vi "test Compile RaF Data.vi"(8 "error in (no error)":errorcluster, 11 "TestCase in":refnum<class "Routing and Faulting Unit Tests.lvclass">) -> (0 "error out":errorcluster, 3 "TestCase out":refnum<class "Routing and Faulting Unit Tests.lvclass">)   [LabVIEW 2017, in "Routing and Faulting Unit Tests.lvclass"]
uses:
  Routing and Faulting Unit Tests.lvclass
  Shared/Communication Configuration.ctl
  Shared/Routing and Faulting Configuration.ctl
  Shared/Routing Channel Configuration.ctl
  Shared/Value-Connections Map.ctl
  Shared/Connection.ctl
  Shared/Alias Mapping.ctl
  Shared/FIFO Indices.ctl
  Shared/Channel States.ctl
  Shared/Routing State.ctl
  Shared/Compiled.Settings.ctl
  Routing and Faulting Unit Tests.lvclass/Routing and Faulting Unit Tests.ctl
  System Explorer/Get Channel Data in By Channel ID (offline).vi
  Scripting/Switch Scripting.lvlib
  Shared/Routing and Faulting Shared.lvlib
  System Explorer/Routing and Faulting System Explorer.lvlib
panel:
  out "Compiled.Settings":T8
  in  "Save?":bool
  out "Output Filename":string
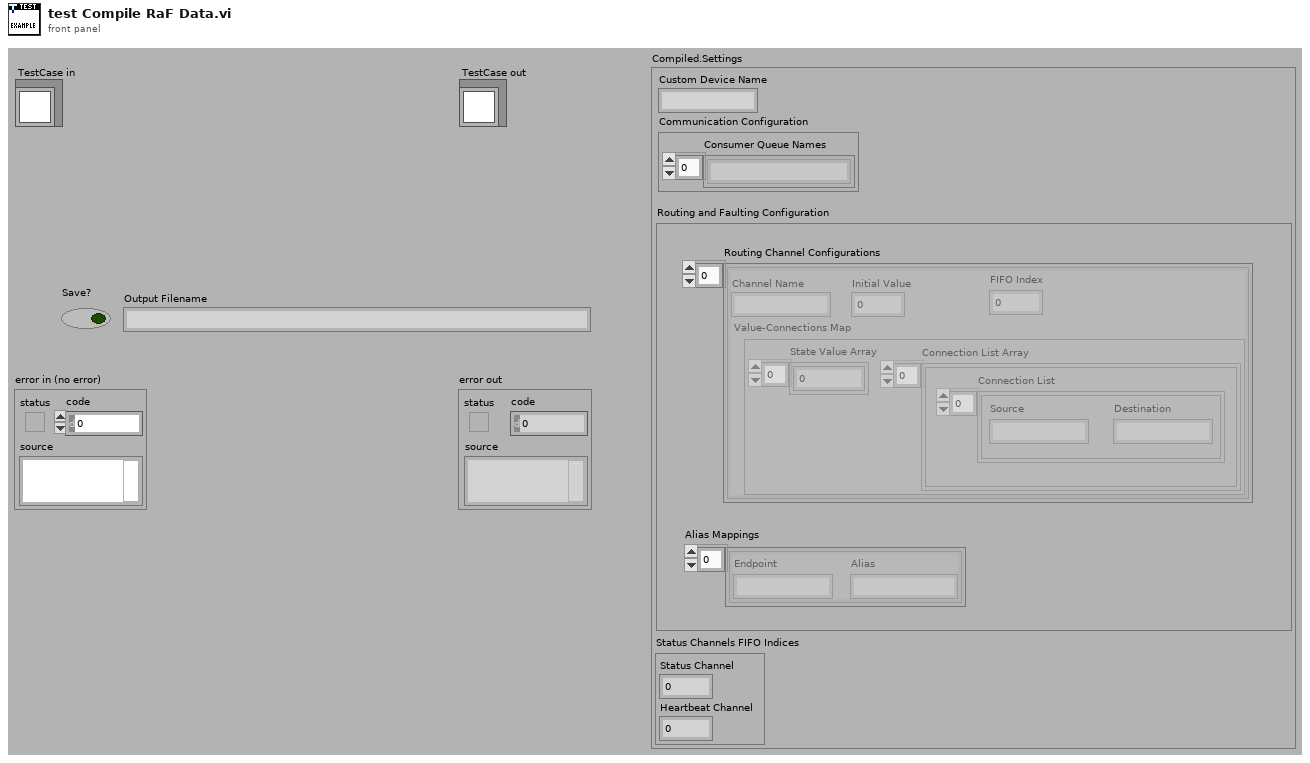
[diagram p1: front panel]
types:
  T1 = typedef "Routing and Faulting Shared.lvlib/Communication Configuration.ctl" = cluster{"Consumer Queue Names":string[]}
  T2 = typedef "Routing and Faulting Shared.lvlib/Routing and Faulting Configuration.ctl" = cluster{"Routing Channel Configurations":T3[], "Alias Mappings":T6[]}
  T3 = typedef "Routing and Faulting Shared.lvlib/Routing Channel Configuration.ctl" = cluster{"Channel Name":string, "Initial Value":dbl, "FIFO Index":i32, "Value-Connections Map":T4}
  T4 = typedef "Routing and Faulting Shared.lvlib/Value-Connections Map.ctl" = cluster{"State Value Array":i32[], "Connection List Array":cluster{"Connection List":T5[]}[]}
  T5 = typedef "Routing and Faulting Shared.lvlib/Connection.ctl" = cluster{"Source":string, "Destination":string}
  T6 = typedef "Routing and Faulting Shared.lvlib/Alias Mapping.ctl" = cluster{"Endpoint":string, "Alias":string}
  T7 = typedef "Routing and Faulting Shared.lvlib/FIFO Indices.ctl" = cluster{"Status Channel":i32, "Heartbeat Channel":i32}
  T8 = cluster{"Custom Device Name":string, "Communication Configuration":T1, "Routing and Faulting Configuration":T2, "Status Channels FIFO Indices":T7}
  T9 = typedef "Routing and Faulting Shared.lvlib/Compiled.Settings.ctl" = cluster{"Custom Device Name":string, "Communication Configuration":T1, "Routing and Faulting Configuration":T2, "Status Channels FIFO Indices":T7}
  T10 = typedef "Routing and Faulting Shared.lvlib/Channel States.ctl" = T11[]
  T11 = typedef "Routing and Faulting Shared.lvlib/Routing State.ctl" = cluster{"Name":string, "Description":string, "Value":i32, "Connection List":T5[]}
  T12 = typedef "Custom Device API.lvlib/Custom Device Item Ref.ctl" = u64
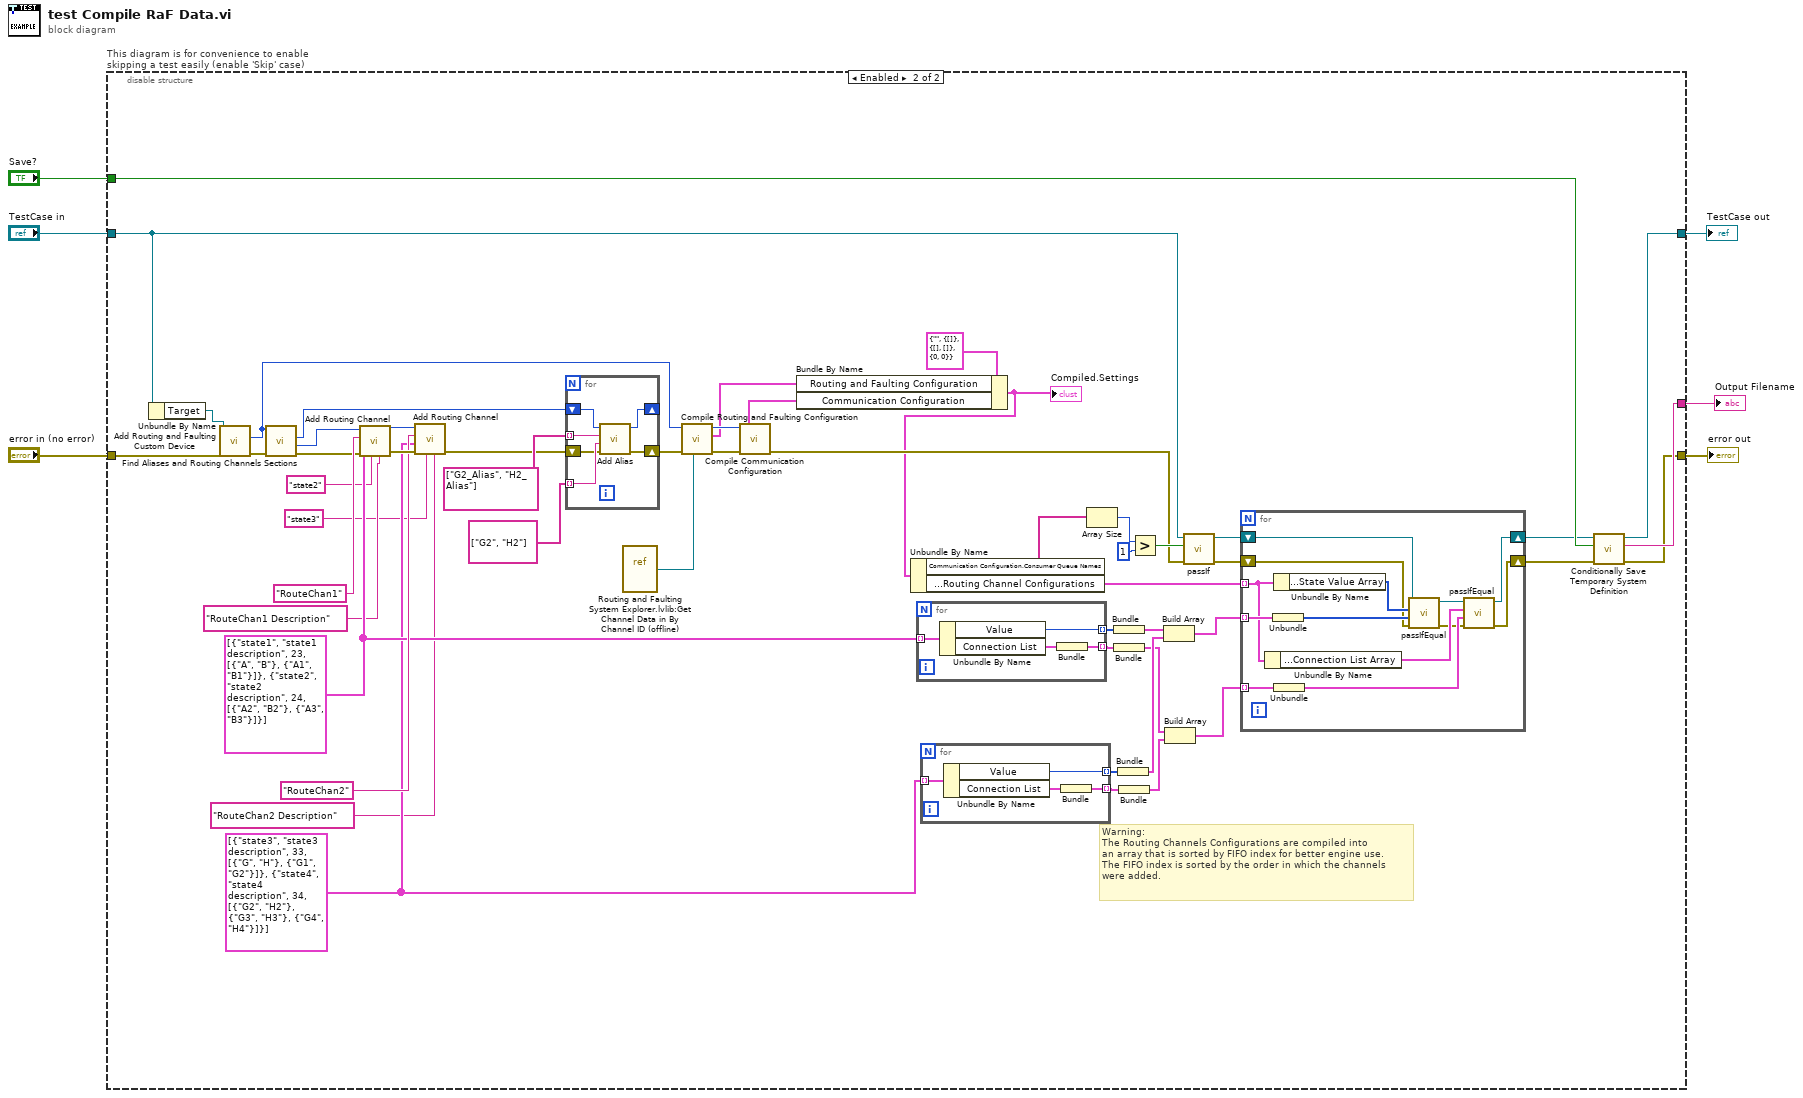
[diagram p0: block diagram]
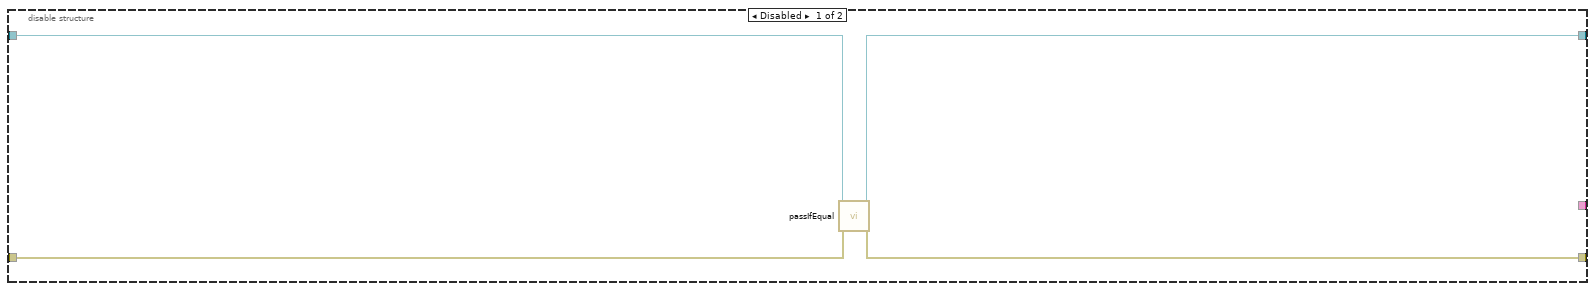
[diagram p2: hidden frame]
diagram:
  n1 = disable-structure "This diagram is for convenience to enable skipping a test easily (enable 'Skip' case)" shown="Enabled" {
    disable-tunnel: "TestCase in" -> [w10 w49]
    disable-tunnel: [w9 w58] -> w3
    disable-tunnel: [w8 w34] -> w5
    disable-tunnel: "error in (no error)" -> [w7 w60]
    disable-tunnel: "Save?" -> [_ w59]
    disable-tunnel: [_ w57] -> w1
    frame Disabled {
      n2 = call-dynamic "passIfEqual.vi"("error in (no error)"=w7, "TestCase in"=w10) -> ("error out"=w8:errorcluster, "TestCase out"=w9:refnum<class "Routing and Faulting Unit Tests.lvclass">)  [unwired: 8 in]
    }
    frame Enabled {
      w28 = T10 [{"Name"="state3", "Description"="state3 description", "Value"=33, "Connection List"=[{"Source"="G", "Destination"="H"}, {"Source"="G1", "Destination"="G2"}]}, {"Name"="state4", "Description"="state4 description", "Value"=34, "Connection List"=[{"Source"="G2", "Destination"="H2"}, {"Source"="G3", "Destination"="H3"}, {"Source"="G4", "Destination"="H4"}]}] ("States and Connections")
      w46 = T10 [{"Name"="state1", "Description"="state1 description", "Value"=23, "Connection List"=[{"Source"="A", "Destination"="B"}, {"Source"="A1", "Destination"="B1"}]}, {"Name"="state2", "Description"="state2 description", "Value"=24, "Connection List"=[{"Source"="A2", "Destination"="B2"}, {"Source"="A3", "Destination"="B3"}]}] ("States and Connections")
      # "Warning: \nThe Routing Channels Configurations are compiled into\nan array that is sorted by FIFO index for better engine use.\nThe FIFO index is sorted by the order in which the channels\nwere added."
      n3 = Unbundle By Name(w49) -> ("Target"=w61:refnum<k24>)
      n4 = call "Add Routing and Faulting Custom Device.vi"("error in (no error)"=w60, "Target in"=w61) -> ("error out"=w63:errorcluster, "Routing and Faulting Custom Device Ref"=w15:T12)  [unwired: 7 in, 1 out]
      n5 = call "Find Aliases and Routing Channels Sections.vi"("error in (no error)"=w63, "Routing and Faulting Custom Device Ref in"=w15) -> ("error out"=w27:errorcluster, "Routing Channels Ref"=w26:T12, "Aliases Ref"=w25:T12)  [unwired: 6 in, 1 out]
      n6 = call "Add Routing Channel.vi"("Description"="RouteChan1 Description", "Initial State"="state2", "error in (no error)"=w27, "State and Connections List"=w46, "Channel Name"="RouteChan1", "Routing Channels Ref in"=w26) -> ("error out"=w56:errorcluster, "Routing Channels Ref out"=w55:T12)  [unwired: 3 in, 1 out]
      n7 = call "Add Routing Channel.vi"("Description"="RouteChan2 Description", "Initial State"="state3", "error in (no error)"=w56, "State and Connections List"=w28, "Channel Name"="RouteChan2", "Routing Channels Ref in"=w55) -> ("error out"=w29:errorcluster)  [unwired: 3 in, 2 out]
      n8 = for {
        shift-right: [w66] -> _
        shift-left: w25 -> [w67]
        tunnel: string[] ["G2_Alias", "H2_Alias"] -> [w69] mode=indexing
        tunnel: string[] ["G2", "H2"] -> [w68] mode=indexing
        shift-right: [w65] -> w14
        shift-left: w29 -> [w64]
        n9 = call "Add Alias.vi"("error in (no error)"=w64, "Endpoint"=w68, "Alias"=w69, "Aliases Ref in"=w67) -> ("error out"=w65:errorcluster, "Aliases Ref out"=w66:T12)  [unwired: 6 in]
      }
      n10 = vi-ref "Routing and Faulting System Explorer.lvlib:Get Channel Data in By Channel ID (offline).vi"() -> (w11:refnum<vi>)
      n11 = call "Compile Routing and Faulting Configuration.vi"("Get Channel Data Refnum"=w11, "error in (no error)"=w14, "Device Ref in"=w15) -> ("error out"=w18:errorcluster, "RaF Configuration"=w16:T2, "Device Ref out"=w19:T12)  [unwired: 6 in]
      n12 = call "Compile Communication Configuration.vi"("error in (no error)"=w18, "Device Ref in"=w19) -> ("error out"=w13:errorcluster, "Communication Configuration"=w17:T1)  [unwired: 7 in, 1 out]
      n13 = Bundle By Name(cluster=T9 {"Custom Device Name"="", "Communication Configuration"={"Consumer Queue Names"=[]}, "Routing and Faulting Configuration"={"Routing Channel Configurations"=[], "Alias Mappings"=[]}, "Status Channels FIFO Indices"={"Status Channel"=0, "Heartbeat Channel"=0}} ("Compiled.Settings.ctl"), "Routing and Faulting Configuration"=w16, "Communication Configuration"=w17) -> (w12:T9)
      "Compiled.Settings" <- w12
      n14 = Unbundle By Name(w12) -> ("Communication Configuration.Consumer Queue Names"=w53:string[], "Routing and Faulting Configuration.Routing Channel Configurations"=w48:T3[])
      n15 = for {
        tunnel: [w77] -> w47 mode=indexing
        tunnel: [w75] -> w43 mode=indexing
        tunnel: w46 -> [w74] mode=indexing
        n16 = Unbundle By Name(w74) -> ("Value"=w77:i32, "Connection List"=w76:T5[])
        n17 = Bundle("Connection List"=w76) -> (w75:cluster{"Connection List":T5[]})  [unwired: 1 in]
      }
      n18 = for {
        tunnel: [w73] -> w45 mode=indexing
        tunnel: [w71] -> w42 mode=indexing
        tunnel: w28 -> [w70] mode=indexing
        n19 = Unbundle By Name(w70) -> ("Value"=w73:i32, "Connection List"=w72:T5[])
        n20 = Bundle("Connection List"=w72) -> (w71:cluster{"Connection List":T5[]})  [unwired: 1 in]
      }
      n21 = Array Size(array=w53) -> (size(s)=w52:i32)
      n22 = Bundle(w47) -> (w41:cluster{i32[]})  [unwired: 1 in]
      n23 = Bundle(w43) -> (w40:cluster{cluster{"Connection List":T5[]}[]})  [unwired: 1 in]
      n24 = Bundle(w45) -> (w44:cluster{i32[]})  [unwired: 1 in]
      n25 = Bundle(w42) -> (w39:cluster{cluster{"Connection List":T5[]}[]})  [unwired: 1 in]
      n26 = Greater?(x=w52, y=1) -> (0:w50:bool)
      n27 = Build Array(w41, w44) -> (w38:cluster{i32[]}[])
      n28 = Build Array(w40, w39) -> (w37:cluster{cluster{"Connection List":T5[]}[]}[])
      n29 = call-dynamic "passIf.vi"("error in (no error)"=w13, "pass"=w50, "TestCase in"=w49) -> ("error out"=w33:errorcluster, "TestCase out"=w36:refnum<class "Routing and Faulting Unit Tests.lvclass">)  [unwired: 7 in]
      n30 = for {
        tunnel: w48 -> [w84] mode=indexing
        tunnel: w38 -> [w90] mode=indexing
        tunnel: w37 -> [w86] mode=indexing
        shift-right: [w81] -> w35
        shift-left: w36 -> [w80]
        shift-right: [w78] -> w32
        shift-left: w33 -> [w79]
        n31 = Unbundle By Name(w84) -> ("Value-Connections Map.Connection List Array"=w87:cluster{"Connection List":T5[]}[])
        n32 = Unbundle(w90) -> (w89:i32[])
        n33 = Unbundle By Name(w84) -> ("Value-Connections Map.State Value Array"=w88:i32[])
        n34 = Unbundle(w86) -> (w85:cluster{"Connection List":T5[]}[])
        n35 = call-dynamic "passIfEqual.vi"("error in (no error)"=w79, "y"=w89, "x"=w88, "TestCase in"=w80) -> ("error out"=w83:errorcluster, "TestCase out"=w82:refnum<class "Routing and Faulting Unit Tests.lvclass">)  [unwired: 6 in]
        n36 = call-dynamic "passIfEqual.vi"("error in (no error)"=w83, "y"=w85, "x"=w87, "TestCase in"=w82) -> ("error out"=w78:errorcluster, "TestCase out"=w81:refnum<class "Routing and Faulting Unit Tests.lvclass">)  [unwired: 6 in]
      }
      n37 = call "Conditionally Save Temporary System Definition.vi"("error in (no error)"=w32, "Save?"=w59, "TestCase in"=w35) -> ("error out"=w34:errorcluster, "filename"=w57:string, "TestCase out"=w58:refnum<class "Routing and Faulting Unit Tests.lvclass">)  [unwired: 6 in]
    }
  }
  "error out" <- w5
  "TestCase out" <- w3
  "Output Filename" <- w1
